vi "VarArray_Get elements.vi"(8 "Error In":errorcluster, 9 "Index Array In":i32[](array[numeric]), 11 "Array In In":variant[](array[variant])) -> (0 "Error Out":errorcluster, 1 "Selected Array Out":variant[](array[variant]))   [LabVIEW 2015]
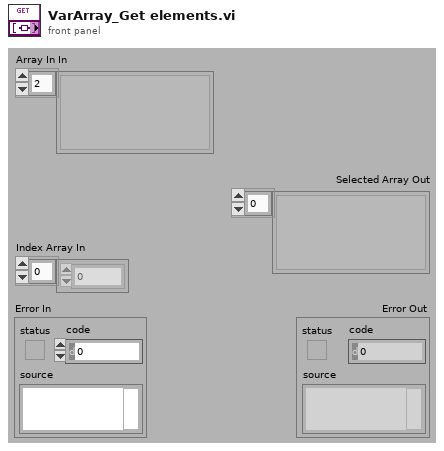
[diagram p1: front panel]
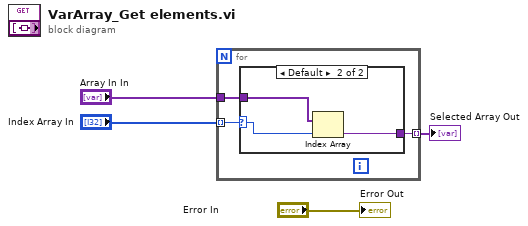
[diagram p0: block diagram]
diagram:
  n1 = for {
    tunnel: "Index Array In" -> [w5] mode=indexing
    tunnel: [w6] -> w2 mode=indexing
    tunnel: "Array In In" -> [w7]
    n2 = case shown="Default" w5 {
      selector: w5 -> [_ w8]
      tunnel: w7 -> [_ w10]
      tunnel: [_ w9] -> w6
      frame -1 {
      }
      frame Default {
        n3 = Index Array(array=w10, index=w8) -> (element=w9:variant)
      }
    }
  }
  "Selected Array Out" <- w2
  "Error Out" <- "Error In"
